vi "fpga_MultiChannel Filtering.vi"(0 "data input":i32, 1 "ARC Constants":T2={"bufsize"=2048, "bufsize-1"=2047, "NChan"=8, "NChan-1"=7, "1/2SymPeriods"=20, "Neg1/2SymPeriods"=-20, "polyOrder-1"=7, "maxDec-1"=24}, 5 "data valid":bool, 7 "filter info":T1 {"coef [I32.2]" format="%#_6f"}, 9 "filter valid":bool, 12 "Ready for output":bool) -> (4 "even-angle signal[I32.3]":fxp<+/-,32,3> format="%.30g", 10 "output valid":bool, 14 "ready for filter":bool)   [LabVIEW 2013, in "NI_EP_Resample_FPGA.lvlib"]
uses:
  <vilib>/addons/Electrical Power/PQ/Resampling/NI_EP_Resample_FPGA.lvlib
  <vilib>/rvi/Emulation/niFpgaSctlEmulationGetInTimedLoop.vi
  <vilib>/rvi/DataTransferAndStorage/Container/Common/niFpgaContainerGetUniqueNameForEmu.vi
  <vilib>/rvi/DataTransferAndStorage/Container/Common/niFpgaContainerSetEmuInfo.vi
  <vilib>/rvi/eio/common/nirviEmuReportErrorAndStop.vi
  <vilib>/rvi/Memory/Memory_Emulation/nirvimemoryEmulation.vi
  <vilib>/rvi/Memory/Memory_Emulation/nirvimemoryFastEmulation.vi
  <vilib>/rvi/Memory/Memory_Emulation/niFpgaMemoryEmulationCacheClearOnFirstRun.vi
  <vilib>/rvi/Memory/Memory_Emulation/nirvimemoryEmulationManagerCache_MakeExclusive.vi
  <vilib>/rvi/Memory/Memory_Emulation/niFpgaMemoryEmulationValidateCache.vi
  <vilib>/rvi/Memory/Memory_Emulation/nirvimemoryEmulationManagerCache_ReleaseExclusive.vi
  <vilib>/rvi/Memory/Memory_Emulation/nirvimemoryEmulationManagerCache_InsertValue.vi
  <vilib>/Utility/error.llb/Clear Errors.vi
  <vilib>/rvi/Memory/Memory_Emulation/nirvimemoryEmulationManagerCache_SetValue.vi
  <vilib>/rvi/Emulation/niFpgaSctlEmulationResourceMgr.vi
  <vilib>/rvi/FIFO/Fifo_Resource/nirvififoEmulationSetSize.vi
  <vilib>/rvi/errors/niFpgaSetErrorForExecOnDevCompSimple.vi
  <vilib>/rvi/Emulation/niFpgaSctlEmulationFifoFullMgr.vi
  <vilib>/rvi/Memory/Memory_Emulation/nirvimemoryEmulationManagerCache_GetValue.vi
  <vilib>/rvi/Arithmetic/AddSubMult/XNode/nirviSatArithmetic.xnode
  <vilib>/rvi/LocalResourceManager/LocalResourceManager.xnode
  <vilib>/rvi/FXPMathLib/basic elements/FxpAddSub/XNode/nifxpmath_AddSub.xnode
  <vilib>/rvi/DataTransferAndStorage/Container/XNode/niFpgaContainer.xnode
  <vilib>/rvi/FXPMathLib/basic elements/FxpDiscreteDelay/XNode/nifxpmath_DiscreteDelay.xnode
  <vilib>/rvi/FXPMathLib/FxpMul/XNode/nifxpmath_Multiplier.xnode
  <vilib>/rvi/FIFO/Fifo_Resource/nirvififoEmulationWrite.vi
  <vilib>/rvi/FIFO/Fifo_Resource/nirvififoEmulationRead.vi
  <vilib>/rvi/FXPMathLib/sim/FxpSim.dll
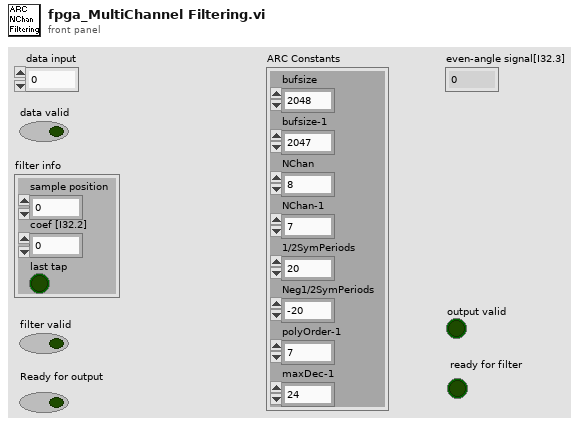
[diagram p1: front panel]
types:
  T1 = cluster{"sample position":u16, "coef [I32.2]":fxp<+/-,32,2>, "last tap":bool}
  T2 = cluster{"bufsize":u16, "bufsize-1":u16, "NChan":u8, "NChan-1":u8, "1/2SymPeriods":i8, "Neg1/2SymPeriods":i8, "polyOrder-1":u8, "maxDec-1":u8}
  T3 = cluster{"mem address":u16, "chan#":u8, "cirbuf ptr":u16}
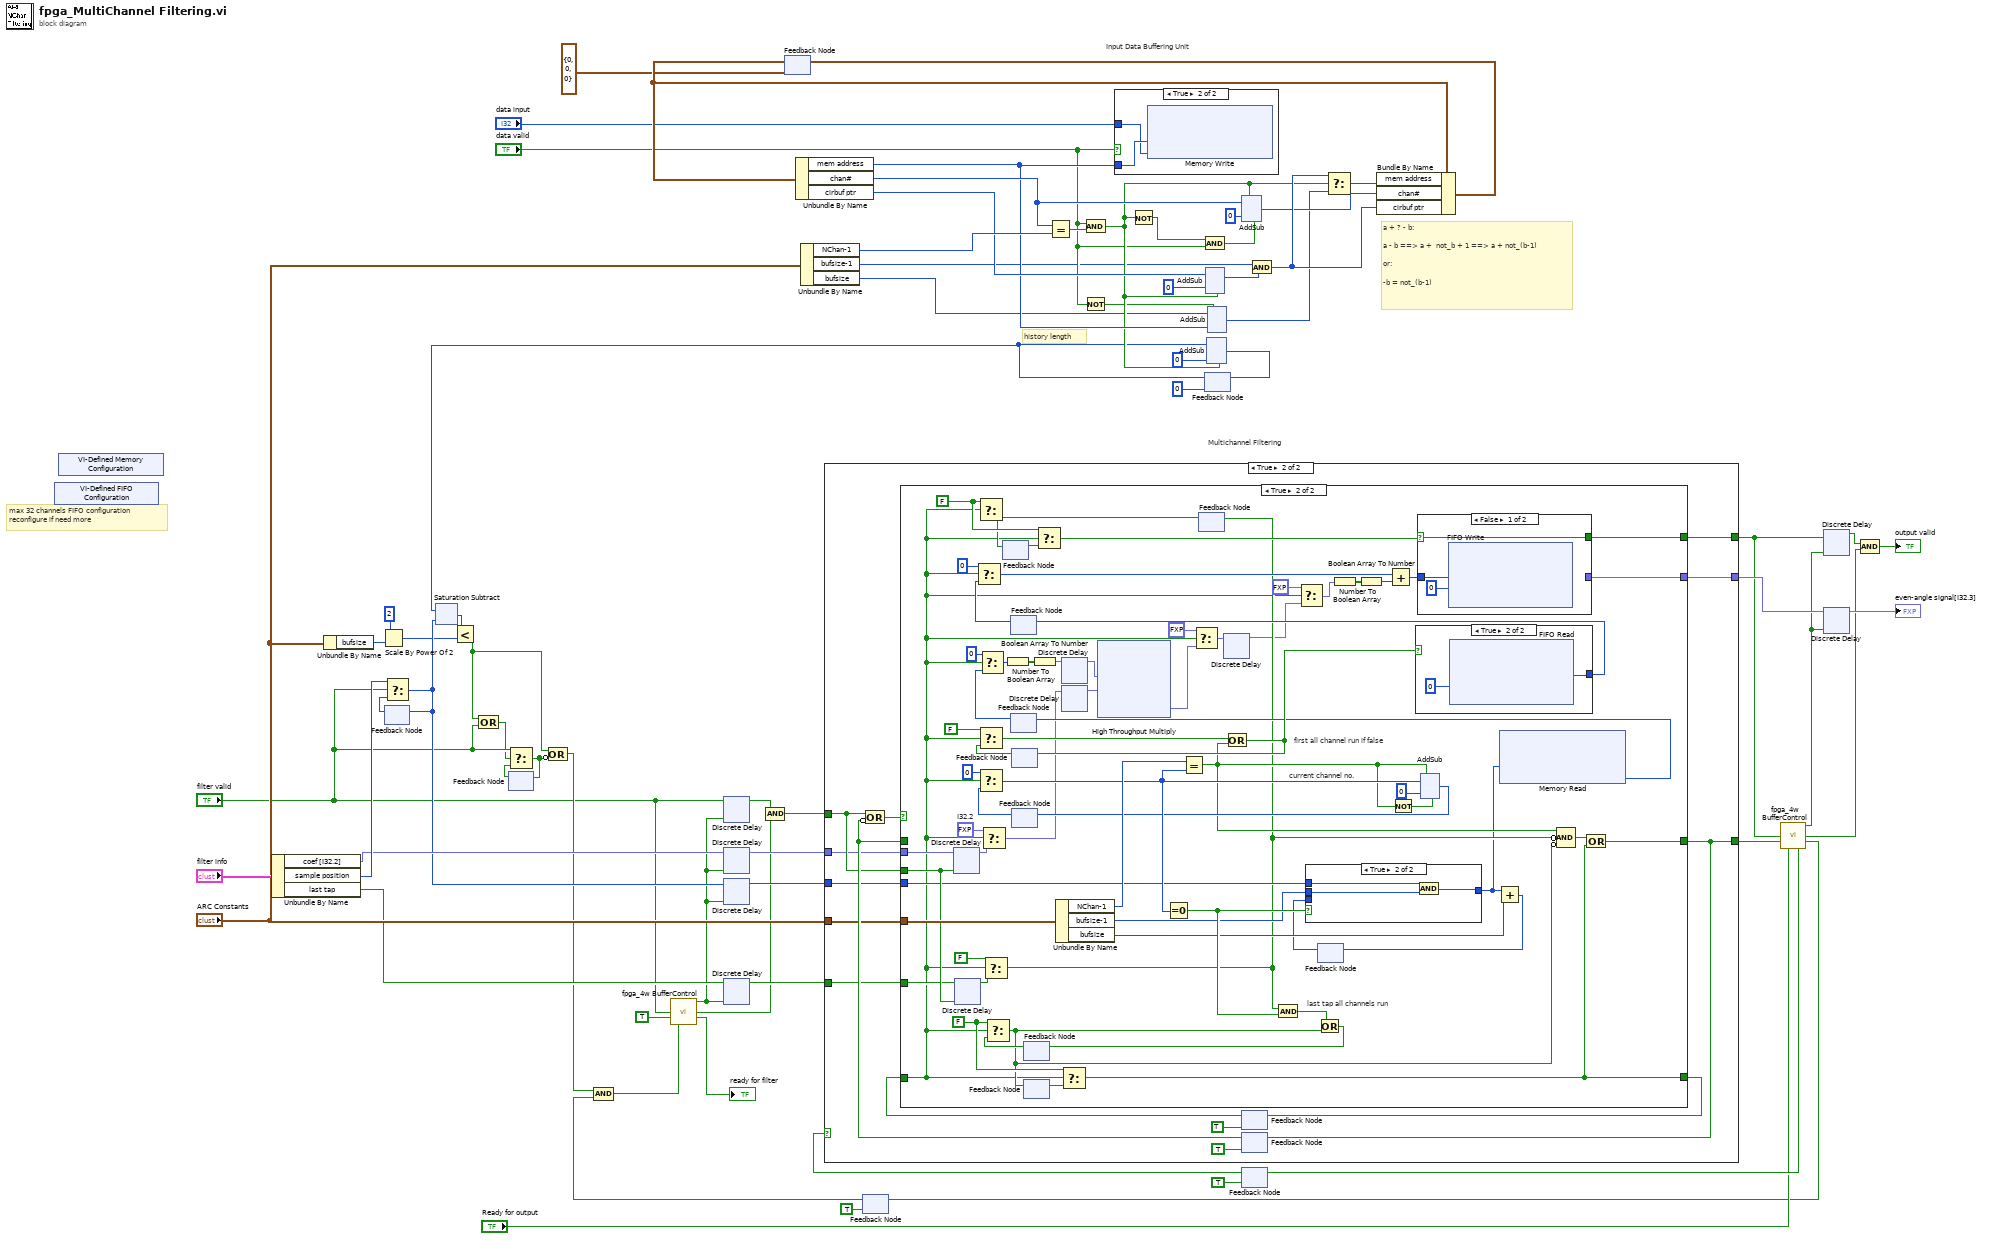
[diagram p0: block diagram]
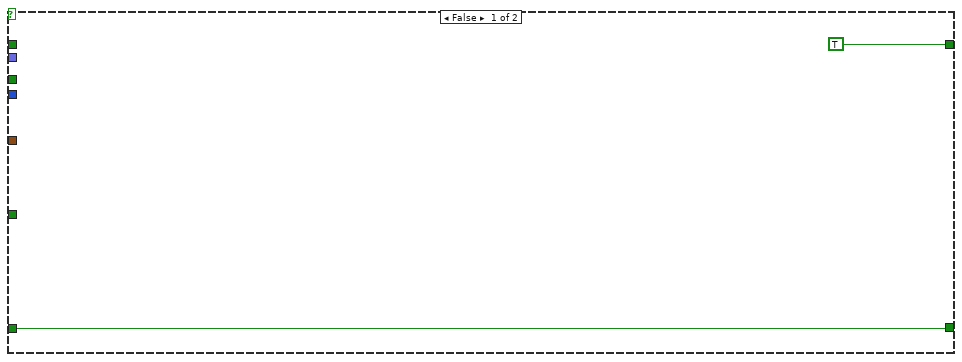
[diagram p4: hidden frame]
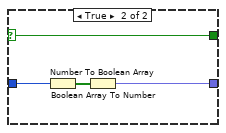
[diagram p5: hidden frame]
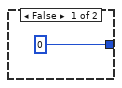
[diagram p7: hidden frame]
diagram:
  # "Multichannel Filtering"
  # "history length"
  # "a + ? - b:\n\na - b ==> a +  not_b + 1 ==> a + not_(b-1)\n\nor:\n\n-b = not_(b-1)"
  # "Input Data Buffering Unit"
  # "max 32 channels FIFO configuration\nreconfigure if need more"
  n1 = xnode "VI-Defined FIFO Configuration"() -> ()  [unwired: 1 out]
  n2 = xnode "VI-Defined Memory Configuration"() -> ()  [unwired: 1 out]
  n3 = Unbundle By Name("filter info") -> ("coef [I32.2]"=w20:fxp<+/-,32,2>, "sample position"=w21:u16, "last tap"=w19:bool)
  n4 = Unbundle By Name("ARC Constants") -> ("bufsize"=w11:u16)
  n5 = Scale By Power Of 2(n=2, x=w11) -> (x*2^n=w12:u16)
  n6 = feedback #1() -> (w37:u16)  [unwired: 1 out]
  n7 = Select(t=w21, s="filter valid", f=w37) -> (s? t:f=w16:u16)
  n8 = feedback-in #1(w16) -> ()
  n9 = feedback #2() -> (w6:bool)  [unwired: 1 in]
  n10 = feedback #3(T3 {"mem address"=0, "chan#"=0, "cirbuf ptr"=0} ("initial address")) -> (w46:T3)
  n11 = Unbundle By Name(w46) -> ("mem address"=w51:u16, "chan#"=w59:u8, "cirbuf ptr"=w54:u16)
  n12 = Unbundle By Name("ARC Constants") -> ("NChan-1"=w60:u8, "bufsize-1"=w40:u16, "bufsize"=w38:u16)
  n13 = feedback #4(TRUE ("ready for input")) -> (w18:bool)
  n14 = Equal?(x=w59, y=w60) -> (x = y?=w63:bool)
  n15 = And(x="data valid", y=w63) -> (x .and. y?=w49:bool)
  n16 = Not(x="data valid") -> (.not. x?=w43:bool)
  n17 = case shown="True" "data valid" {
    tunnel: w51 -> [_ w71]
    tunnel: "data input" -> [_ w70]
    frame False {
    }
    frame True {
      n18 = xnode ("Memory Write")("Address"=w71, "Data"=w70) -> ()  [unwired: 1 in, 1 out]
    }
  }
  n19 = Not(x=w49) -> (.not. x?=w56:bool)
  n20 = And(x=w56, y="data valid") -> (x .and. y?=w57:bool)
  n21 = feedback #5(u16 0 ("s")) -> (w15:u16)
  n22 = xnode "Saturation Subtract"("x"=w15, "y"=w16) -> ("x-y"=w23:u16)
  n23 = Less?(x=w23, y=w12) -> (x < y?=w3:bool)
  n24 = Compound Arithmetic op=OR(w3, "filter valid") -> (w4:bool)
  n25 = Select(t="filter valid", s=w4, f=w6) -> (s? t:f=w2:bool)
  n26 = feedback-in #2(w2) -> ()
  n27 = Compound Arithmetic op=OR(w3, invert w2) -> (w9:bool)
  n28 = Compound Arithmetic op=AND(w9, w18) -> (w1:bool)
  n29 = call <vilib>:"fpga_4w BufferControl.vi"("DR"="filter valid", "RFI"=TRUE, "RFO"=w1) -> ("buff enable"=w8:bool, "output valid"=w14:bool, "ready for input"=→"ready for filter":bool)  [unwired: 9 in, 1 out]
  n30 = xnode "Discrete Delay"("D"="filter valid", "enable"=w8) -> ("Q"=w7:bool)
  n31 = xnode "Discrete Delay"("D"=w20, "enable"=w8) -> ("Q"=w27:fxp<+/-,32,2>)
  n32 = xnode "Discrete Delay"("D"=w16, "enable"=w8) -> ("Q"=w26:u16)
  n33 = xnode "Discrete Delay"("D"=w19, "enable"=w8) -> ("Q"=w25:bool)
  n34 = Compound Arithmetic op=AND(w7, w14) -> (w29:bool)
  n35 = xnode "AddSub"("x"=w54, "y"=u16 0, "carry-in"=w49) -> ("s"=w52:u16)  [unwired: 1 out]
  n36 = xnode "AddSub"("x"=w15, "y"=u16 0, "carry-in"=w49) -> ("s"=w44:u16)  [unwired: 1 out]
  n37 = feedback-in #5(w44) -> ()
  n38 = xnode "AddSub"("x"=w38, "y"=w51, "use zero instead of x"=w43) -> ("s"=w50:u16)  [unwired: 1 out]
  n39 = xnode "AddSub"("x"=w59, "y"=u8 0, "carry-in"=w57, "use zero instead of x"=w49) -> ("s"=w55:u8)  [unwired: 1 out]
  n40 = feedback #6(TRUE ("logic enable")) -> (w68:bool)
  n41 = case shown="True" w68 {
    tunnel: w29 -> [_ w83]
    tunnel: "ARC Constants" -> [_ w82]
    tunnel: w27 -> [_ w81]
    tunnel: w25 -> [_ w80]
    tunnel: [_ w77] -> w32
    tunnel: [_ w78] -> w31
    tunnel: [_ w76] -> w65
    tunnel: w26 -> [_ w75]
    frame False {
    }
    frame True {
      n42 = feedback #7(TRUE) -> (w79:bool)
      n43 = feedback #8(TRUE) -> (w84:bool)
      n44 = Compound Arithmetic op=OR(w83, invert w84) -> (w73:bool)
      n45 = case shown="True" w73 {
        tunnel: w79 -> [w87 w88]
        tunnel: [TRUE w99] -> w78
        tunnel: [w87 w100] -> w85
        tunnel: w84 -> [_ _]
        tunnel: w83 -> [_ w109]
        tunnel: w82 -> [_ w110]
        tunnel: w81 -> [_ w108]
        tunnel: w80 -> [_ w107]
        tunnel: [_ w106] -> w76
        tunnel: [_ w105] -> w77
        tunnel: w75 -> [_ w104]
        frame False {
        }
        frame True {
          w112 = FALSE
          w122 = fxp<+/-,32,2> 0.0  # I32.2
          w139 = FALSE
          # "last tap all channels run"
          # "current channel no."
          # "first all channel run if false"
          n46 = xnode "Discrete Delay"("D"=w108, "enable"=w109) -> ("Q"=w117:fxp<+/-,32,2>)
          n47 = xnode "Discrete Delay"("D"=w107, "enable"=w109) -> ("Q"=w115:bool)
          n48 = Select(t=w122, s=w88, f=w117) -> (s? t:f=w102:fxp<+/-,32,2>)
          n49 = Select(t=FALSE, s=w88, f=w115) -> (s? t:f=w97:bool)
          n50 = feedback #9() -> (w137:bool)  [unwired: 1 out]
          n51 = feedback #10() -> (w133:i32)  [unwired: 1 out]
          n52 = Select(t=0, s=w88, f=w133) -> (s? t:f=w132:i32)
          n53 = feedback #11() -> (w131:i32)  [unwired: 1 out]
          n54 = Select(t=0 ("f"), s=w88, f=w131) -> (s? t:f=w149:i32)
          n55 = Number To Boolean Array(number=w149) -> (Boolean array=w148:bool[])
          n56 = feedback #12() -> (w128:bool)  [unwired: 1 out]
          n57 = Select(t=FALSE, s=w88, f=w128) -> (s? t:f=w127:bool)
          n58 = feedback #13() -> (w123:u8)  [unwired: 1 out]
          n59 = Select(t=u8 0 ("nextChan"), s=w88, f=w123) -> (s? t:f=w125:u8)
          n60 = feedback #14() -> (w113:bool)  [unwired: 1 out]
          n61 = Select(t=w112, s=w88, f=w113) -> (s? t:f=w96:bool)
          n62 = feedback-in #15(w96) -> ()
          n63 = feedback #15() -> (w111:bool)  [unwired: 1 out]
          n64 = Boolean Array To Number(Boolean array=w148) -> (number=w147:fxp<+/-,32,1>)
          n65 = Select(t=w139, s=w88, f=w137) -> (s? t:f=w136:bool)
          n66 = Unbundle By Name(w110) -> ("NChan-1"=w154:u8, "bufsize-1"=w120:u16, "bufsize"=w119:u16)
          n67 = xnode "Discrete Delay"("D"=w147) -> ("Q"=w143:fxp<+/-,32,1>)
          n68 = xnode "Discrete Delay"("D"=w102) -> ("Q"=w150:fxp<+/-,32,2>)
          n69 = Select(t=w112, s=w88, f=w111) -> (s? t:f=w100:bool)
          n70 = xnode "High Throughput Multiply"("x"=w143, "y"=w150) -> ("x*y"=w92:fxp<+/-,32,3>)
          n71 = Equal To 0?(x=w125) -> (x = 0?=w152:bool)
          n72 = Equal?(x=w154, y=w125) -> (x = y?=w98:bool)
          n73 = Select(t=fxp<+/-,32,3> 0.0 ("x*y"), s=w88, f=w92) -> (s? t:f=w94:fxp<+/-,32,3>)
          n74 = feedback-in #16(w97) -> ()
          n75 = feedback #16() -> (w140:bool)  [unwired: 1 out]
          n76 = Select(t=w139, s=w88, f=w140) -> (s? t:f=w138:bool)
          n77 = feedback-in #9(w138) -> ()
          n78 = xnode "Discrete Delay"("D"=w94) -> ("Q"=w90:fxp<+/-,32,3>)
          n79 = Or(x=w127, y=w98) -> (x .or. y?=w129:bool)
          n80 = feedback-in #12(w129) -> ()
          n81 = And(x=w97, y=w152) -> (x .and. y?=w144:bool)
          n82 = Select(t=fxp<+/-,32,3> 0.0 ("Q"), s=w88, f=w90) -> (s? t:f=w91:fxp<+/-,32,3>)
          n83 = Or(x=w144, y=w96) -> (x .or. y?=w114:bool)
          n84 = feedback-in #14(w114) -> ()
          n85 = feedback #17() -> (w118:u16)  [unwired: 1 out]
          n86 = case shown="True" w152 {
            tunnel: w118 -> [w211 _]
            tunnel: [w211 w214] -> w95
            tunnel: w120 -> [_ w213]
            tunnel: w104 -> [_ w212]
            frame False {
            }
            frame True {
              n87 = And(x=w212, y=w213) -> (x .and. y?=w214:u16)
            }
          }
          n88 = Number To Boolean Array(number=w91) -> (Boolean array=w146:bool[])
          n89 = Boolean Array To Number(Boolean array=w146) -> (number=w145:i32)
          n90 = Add(x=w132, y=w145) -> (x+y=w142:i32)
          n91 = Not(x=w98) -> (.not. x?=w151:bool)
          n92 = case shown="True" w129 {
            tunnel: [0 ("Element") w217] -> w134
            frame False {
            }
            frame True {
              n93 = xnode ("FIFO Read")("Timeout"=0 ("Timeout (-1 for no timeout)")) -> ("Element"=w217:i32)  [unwired: 1 in, 2 out]
            }
          }
          n94 = feedback-in #10(w134) -> ()
          n95 = case shown="False" w136 {
            selector: w136 -> [w204 w207]
            tunnel: w142 -> [w205 w210]
            tunnel: [_ w208] -> w106
            tunnel: [w204 w207] -> w105
            frame False {
              n96 = xnode ("FIFO Write")("Element"=w205, "Timeout"=0 ("Timeout (-1 for no timeout)")) -> ()  [unwired: 1 in, 2 out]
            }
            frame True {
              n97 = Number To Boolean Array(number=w210) -> (Boolean array=w209:bool[])
              n98 = Boolean Array To Number(Boolean array=w209) -> (number=w208:fxp<+/-,32,3>)
            }
          }
          n99 = xnode "AddSub"("x"=w125, "y"=u8 0, "carry-in"=w151, "use zero instead of x"=w98) -> ("s"=w124:u8)  [unwired: 1 out]
          n100 = feedback-in #13(w124) -> ()
          n101 = Add(x=w95, y=w119) -> (x+y=w121:u16)
          n102 = feedback-in #17(w121) -> ()
          n103 = xnode ("Memory Read")("Address"=w95) -> ("Data"=w103:i32)  [unwired: 1 in, 1 out]
          n104 = feedback-in #11(w103) -> ()
          n105 = Compound Arithmetic op=AND(w98, invert w97, invert w96) -> (w101:bool)
          n106 = Compound Arithmetic op=OR(w101, w100) -> (w99:bool)
        }
      }
      n107 = feedback-in #7(w85) -> ()
      n108 = feedback-in #8(w78) -> ()
    }
  }
  n109 = And(x=w40, y=w52) -> (x .and. y?=w61:u16)
  n110 = Select(t=w61, s=w49, f=w50) -> (s? t:f=w62:u16)
  n111 = Bundle By Name(cluster=w46, "mem address"=w62, "chan#"=w55, "cirbuf ptr"=w61) -> (w47:T3)
  n112 = feedback-in #3(w47) -> ()
  n113 = call <vilib>:"fpga_4w BufferControl.vi"("DR"=w32, "RFI"=w31, "RFO"="Ready for output") -> ("buff enable"=w34:bool, "output valid"=w13:bool, "ready for input"=w28:bool, "logic enable"=w69:bool)  [unwired: 9 in]
  n114 = feedback-in #4(w28) -> ()
  n115 = feedback-in #6(w69) -> ()
  n116 = xnode "Discrete Delay"("D"=w32, "enable"=w34) -> ("Q"=w35:bool)
  n117 = xnode "Discrete Delay"("D"=w65, "enable"=w34) -> ("Q"=→"even-angle signal[I32.3]":fxp<+/-,32,3>)
  n118 = Compound Arithmetic op=AND(w35, w13) -> (→"output valid":bool)
